vi "Read Lidar.vi"(8 "error in (no error)":errorcluster, 9 "clustIn":cluster{"[0]":u32, "[1]":u32}[](array[cluster]), 11 "SerialPortRef":T1) -> (0 "error out":errorcluster, 1 "clustOut":cluster{"[0]":u32, "[1]":u32}[](array[cluster]), 3 "SerialPortRef":T1)   [LabVIEW 2013]
uses:
  <vilib>/Rock Robotics/WPI/SerialPort/WPI_SerialPortRef.ctl
panel:
  out "Packet":i16[][](array[numeric])
  out "Distance":i16[][](array[numeric])
  out "number":i16
  out "Corrected Packet Number":i16
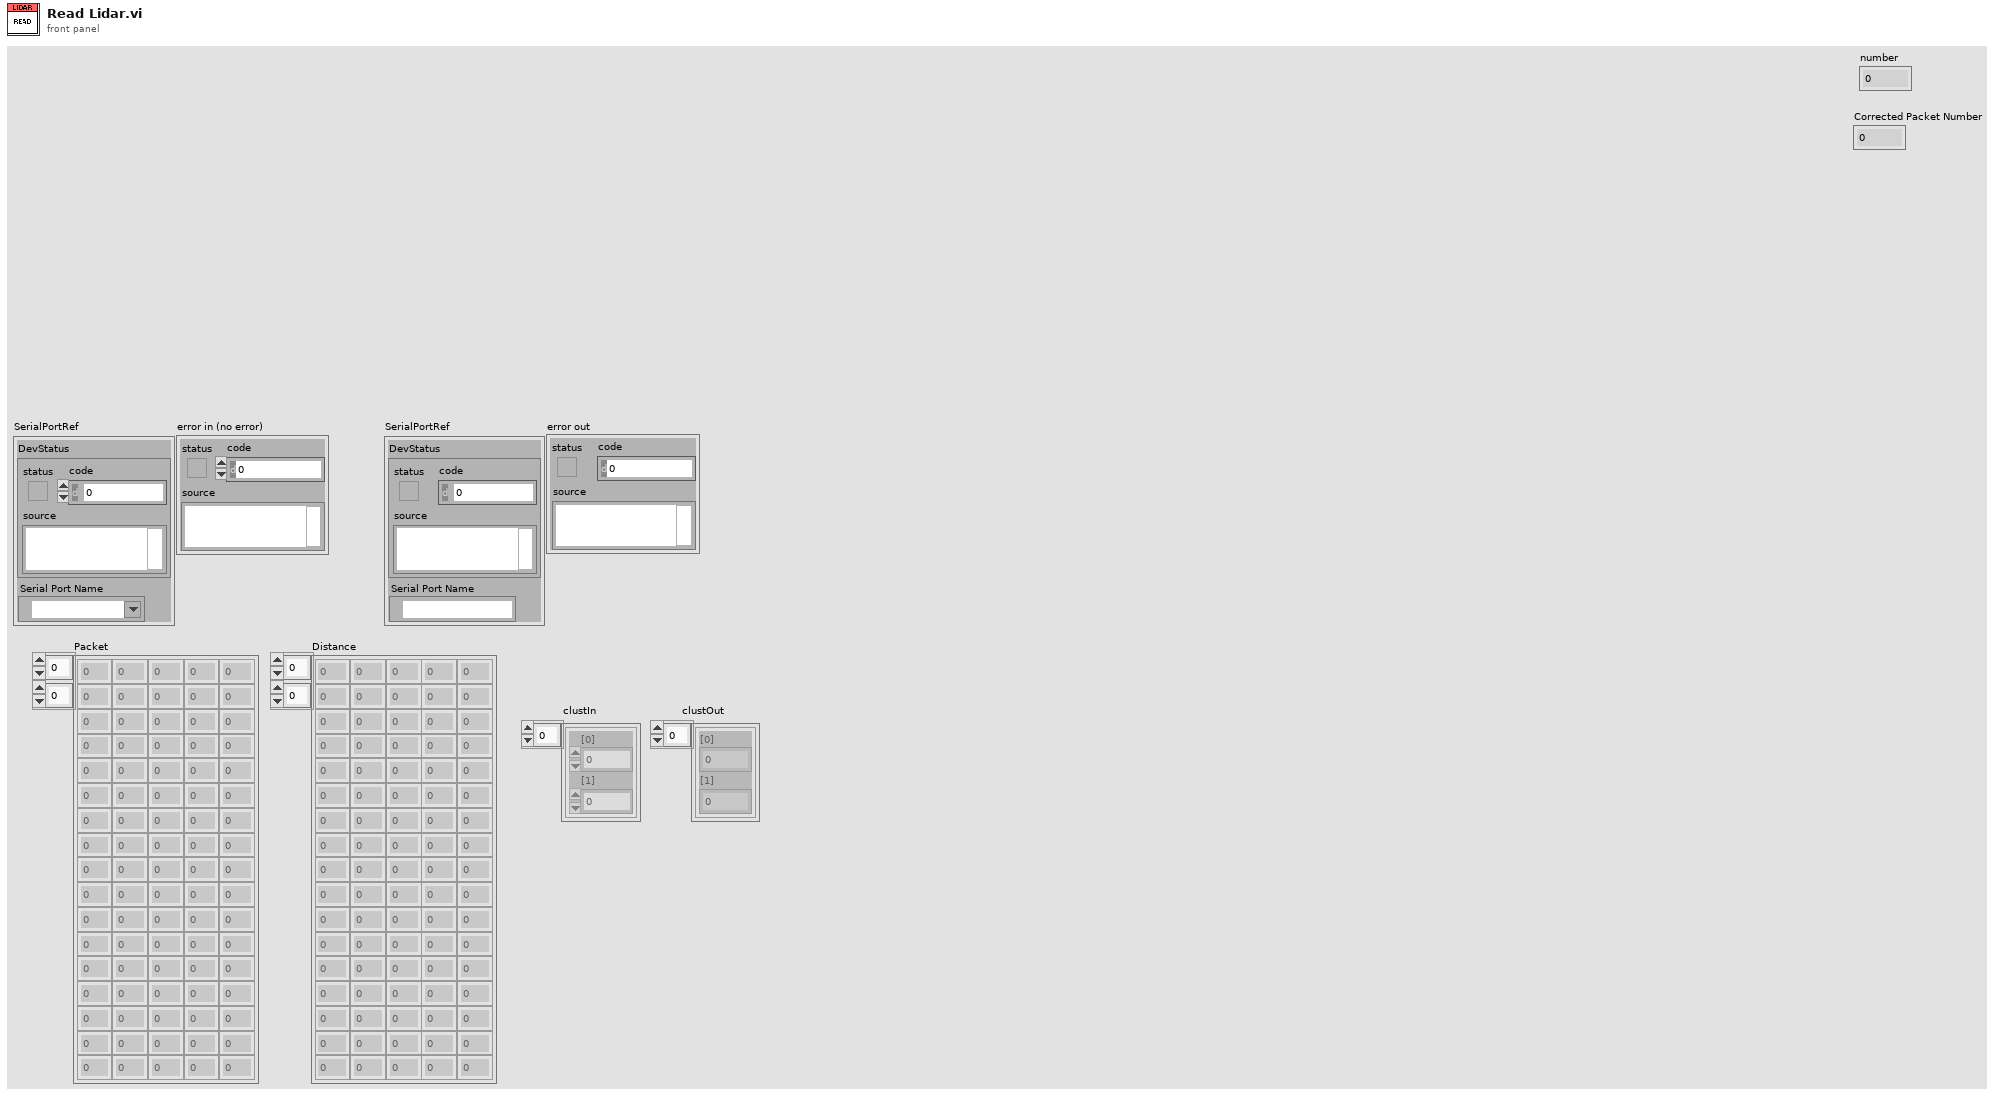
[diagram p1: front panel]
types:
  T1 = typedef "WPI_SerialPortRef.ctl" = cluster{"DevStatus":errorcluster, "Serial Port Name":refnum<visa-resource-name>}
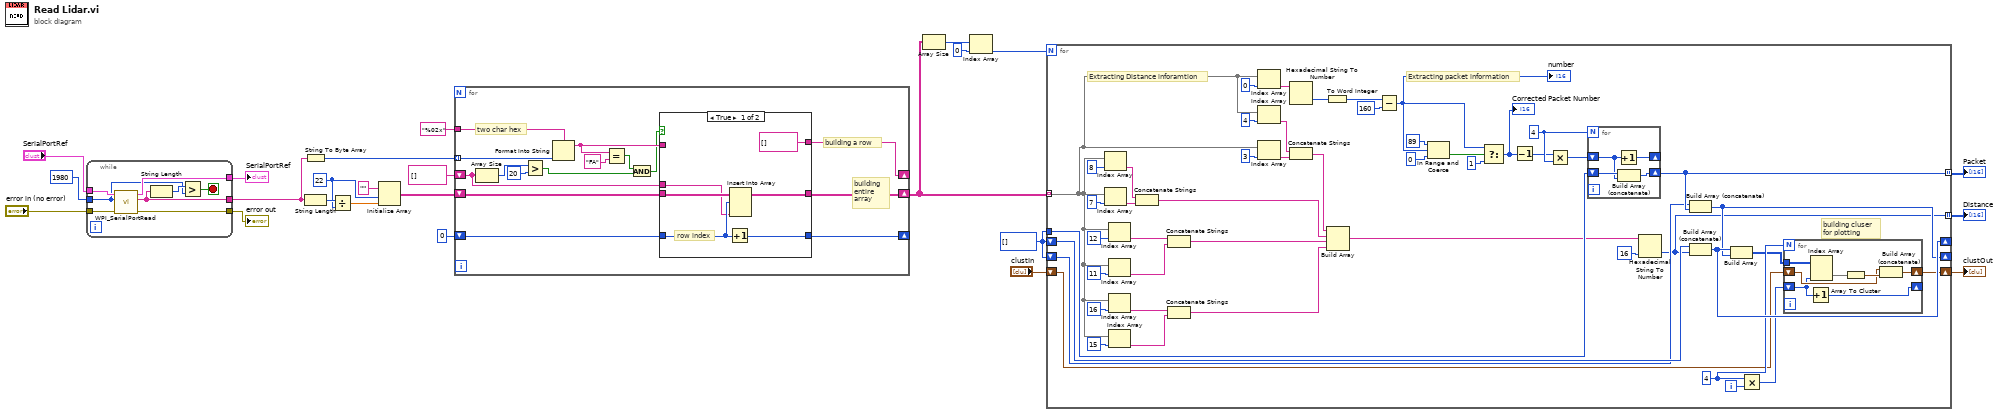
[diagram p0: block diagram]
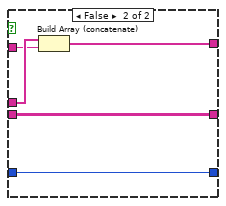
[diagram p2: hidden frame]
diagram:
  w9 = i16[] []
  w19 = 22 ("dimension size")
  n1 = while {
    tunnel: u32 1980 ("Num Bytes to Read") -> [w25]
    tunnel: "SerialPortRef" -> [w32]
    tunnel: "error in (no error)" -> [w31]
    tunnel: [w28] -> w12
    tunnel: [w30] -> w11
    tunnel: [w29] -> w10
    stop <- w27 stop-if-true
    n2 = call <vilib>:"WPI_SerialPortRead.vi"("error in (no error)"=w31, "Num Bytes to Read"=w25, "SerialPortRef"=w32) -> ("error out"=w29:errorcluster, "Buffer"=w28:string, "SerialPortRef"=w30:T1)  [unwired: 6 in]
    n3 = String Length(string=w28) -> (length=w26:i32)
    n4 = Greater?(x=w26, y=w25) -> (0:w27:bool)
  }
  "SerialPortRef" <- w11
  "error out" <- w10
  n5 = String To Byte Array(string=w12) -> (unsigned byte array=w14:u8[])
  n6 = String Length(string=w12) -> (length=w20:i32)
  n7 = Divide(x=w20, y=w19) -> (x/y=w21:dbl)
  n8 = Initialize Array("" ("resulting string"), w19, w21) -> (w16:string[][])
  n9 = for {
    tunnel: "%02x" ("format string") -> [w47]
    tunnel: w14 -> [w46] mode=indexing
    shift-right: [w41] -> _
    shift-left: 0 -> [w42]
    shift-right: [w40] -> w1
    shift-left: w16 -> [w43]
    shift-right: [w39] -> _
    shift-left: string[] [] -> [w36]
    # "building entire\narray"
    # "building a row"
    # "two char hex"
    n10 = Array Size(array=w36) -> (size(s)=w35:i32)
    n11 = Greater?(x=w35, y=20) -> (0:w37:bool)
    n12 = Format Into String(format string=w47, w46) -> (resulting string=w45:string)  [unwired: 2 in, 1 out]
    n13 = Equal?(x=w45, y="FA" ("element")) -> (x = y?=w33:bool)
    n14 = And(x=w33, y=w37) -> (x .and. y?=w38:bool)
    n15 = case shown="True" w38 {
      tunnel: w45 -> [_ w55]
      tunnel: w43 -> [w51 w57]
      tunnel: w42 -> [w52 w58]
      tunnel: [w53 w58] -> w41
      tunnel: [w50 w57] -> w40
      tunnel: w36 -> [w48 w56]
      tunnel: [string[] [] w54] -> w39
      frame True {
        # "row index"
        n16 = Increment(x=w52) -> (x+1=w53:i32)
        n17 = Insert Into Array(array=w51, index (row)=w52, new element=w48) -> (w50:string[][])  [unwired: 1 in]
      }
      frame False {
        n18 = Build Array (concatenate)(w56, w55) -> (w54:string[])
      }
    }
  }
  n19 = Array Size(array=w1) -> (size(s)=w2:i32[])
  n20 = Index Array(array=w2, index=0) -> (element=w7:i32)
  n21 = for {
    N: w7 -> [_]
    tunnel: w1 -> [w74] mode=indexing
    tunnel: [w72] -> w8 mode=indexing
    tunnel: [w91] -> w4 mode=indexing
    tunnel: w9 -> [w95]
    shift-right: [w90] -> _
    shift-left: w9 -> [w93]
    shift-right: [w89] -> _
    shift-left: w9 -> [w88]
    shift-right: [w84] -> w5
    shift-left: "clustIn" -> [w83]
    i -> [w82]
    w87 = 4
    w98 = i16 4 ("y")
    # "building cluser\nfor plotting"
    # "Extracting packet information"
    # "Extracting Distance inforamtion"
    n22 = Index Array(array=w74, index=8) -> (element=w64:string)
    n23 = Index Array(array=w74, index=7) -> (element=w63:string)
    n24 = Index Array(array=w74, index=12) -> (element=w62:string)
    n25 = Index Array(array=w74, index=11) -> (element=w61:string)
    n26 = Index Array(array=w74, index=16) -> (element=w60:string)
    n27 = Index Array(array=w74, index=15) -> (element=w59:string)
    n28 = Concatenate Strings(w64, w63) -> (w70:string)
    n29 = Concatenate Strings(w62, w61) -> (w69:string)
    n30 = Concatenate Strings(w60, w59) -> (w68:string)
    n31 = Index Array(array=w74, index=0) -> (element=w103:string)
    n32 = Index Array(array=w74, index=4) -> (element=w66:string)
    n33 = Index Array(array=w74, index=3) -> (element=w65:string)
    n34 = Hexadecimal String To Number(string=w103) -> (number=w81:u32)  [unwired: 2 in, 1 out]
    n35 = Concatenate Strings(w66, w65) -> (w71:string)
    n36 = To Word Integer(number=w81) -> (16bit integer=w80:i16)
    n37 = Build Array(w71, w70, w69, w68) -> (w67:string[])
    n38 = Subtract(x=w80, y=i16 160) -> (x-y=w96:i16)
    "number" <- w96
    n39 = In Range and Coerce(upper limit=i16 89, x=w96, lower limit=i16 0) -> (In Range?=w100:bool)  [unwired: 1 out]
    n40 = Select(t=w96, s=w100, f=i16 1) -> (s? t:f=w94:i16)
    "Corrected Packet Number" <- w94
    n41 = Decrement(x=w94) -> (x-1=w97:i16)
    n42 = Multiply(x=w97, y=w98) -> (x*y=w99:i16)
    n43 = for {
      N: w98 -> [_]
      shift-right: [w118] -> w91
      shift-left: w95 -> [w119]
      shift-right: [w116] -> _
      shift-left: w99 -> [w117]
      n44 = Increment(x=w117) -> (x+1=w116:i16)
      n45 = Build Array (concatenate)(w119, w117) -> (w118:i16[])
    }
    n46 = Hexadecimal String To Number(string=w67, default (0uL)=u32 16 ("default (0 U32)")) -> (number=w72:u32[])  [unwired: 1 in, 1 out]
    n47 = Build Array (concatenate)(w88, w91) -> (w89:i16[])
    n48 = Build Array (concatenate)(w93, w72) -> (w90:u32[])
    n49 = Build Array(w90, w89) -> (w85:u32[][])
    n50 = Multiply(x=w87, y=w82) -> (x*y=w86:i32)
    n51 = for {
      N: w87 -> [_]
      tunnel: w85 -> [w115]
      shift-right: [w110] -> _
      shift-left: w86 -> [w109]
      shift-right: [w112] -> w84
      shift-left: w83 -> [w111]
      n52 = Increment(x=w109) -> (x+1=w110:i32)
      n53 = Index Array(array=w115, index (col)=w109) -> (element=w114:u32[])  [unwired: 1 in]
      n54 = Array To Cluster(array=w114) -> (cluster=w113:cluster{"[0]":u32, "[1]":u32})
      n55 = Build Array (concatenate)(w111, w113) -> (w112:cluster{"[0]":u32, "[1]":u32}[])
    }
  }
  "Distance" <- w8
  "Packet" <- w4
  "clustOut" <- w5
